vi "ziExample-CNT.vi"() -> ()   [LabVIEW 2009]
doc: "Control a Zurich instrument device via the LabOne Labview API. \nRequirements: Zurich Instruments MFLI, HF2 or UHFLI \nThe example streams the counter data of a trigger input.\n\n© Zurich Instruments AG, www.zhinst.com"
uses:
  <instrlib>/Zurich Instruments LabOne/Public/Configure/ziSetValueDoubleArray.vi
  <instrlib>/Zurich Instruments LabOne/Public/Utility/ziTicksToS_vector.vi
  <instrlib>/Zurich Instruments LabOne/Public/Data/ziGetEventCntSample.vi
  <instrlib>/Zurich Instruments LabOne/Zurich Instruments LabOne.lvlib
panel:
  out "data":cluster{"Timestamp(s)":dbl[], u32[]}
  out "All Values (V)":cluster{"Timestamp(s)":dbl[], i32[]}(graph)
  out "Error Out":errorcluster
  in  "Address":string="DEV"
  out "Selected Device":string
  out "Unexpected Node":string[](array[string])
  in  "stop":bool=TRUE
  # "ziExample-CNT.vi\nRequirements:  UHFLI + CNT Option\nsee block diagram for VI description"
  # "Tested Instruments:\n- UHF"
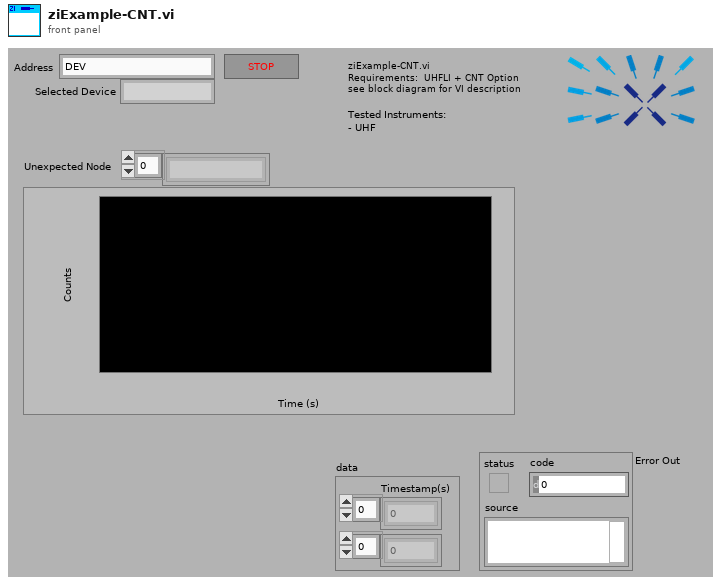
[diagram p1: front panel]
types:
  T1 = typedef "Zurich Instruments LabOne.lvlib/ziTypeHandle.ctl" = cluster{"handleValid":bool, "Conn":u64, "Path Prefix":string, "Handle":u64, "Connected":bool, "Clockbase(s)":dbl}
  T2 = typedef "Zurich Instruments LabOne.lvlib/ziTypeCounterSample.ctl" = cluster{"Timestamps (ticks)":u64[], "Counter":i32[], "Trigger":u32[]}
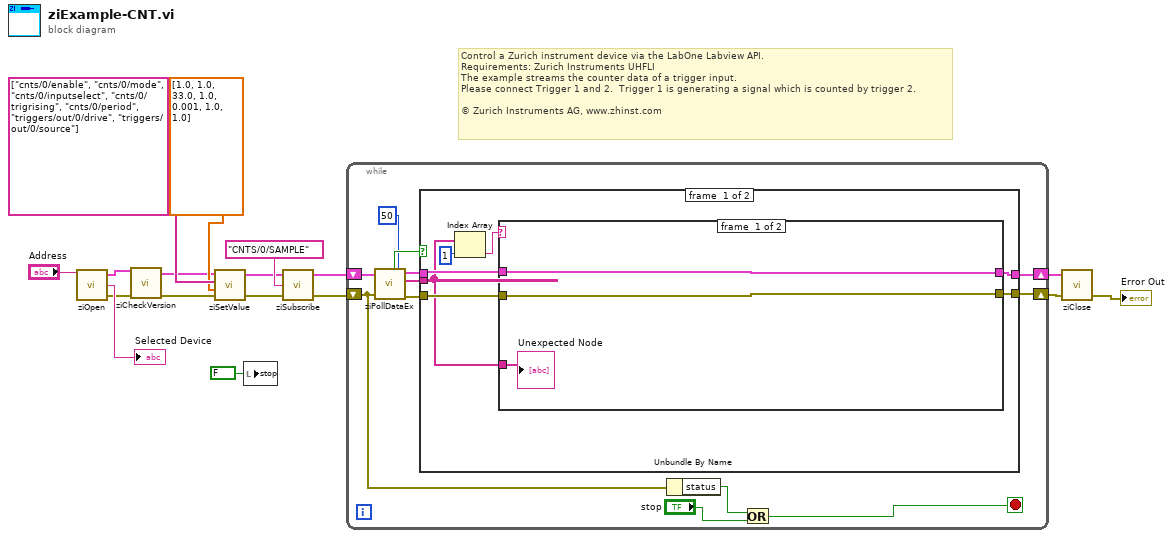
[diagram p0: block diagram]
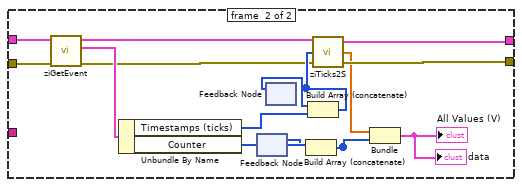
[diagram p2: hidden frame]
diagram:
  # "Control a Zurich instrument device via the LabOne Labview API. \nRequirements: Zurich Instruments UHFLI  \nThe example streams the counter data of a trigger input.\nPlease connect Trigger 1 and 2.  Trigger 1 is generating a signal which is counted by trigger 2.\n\n© Zurich Instruments AG, www.zhinst.com"
  n1 = call <instrlib>:"ziOpen.vi"("Address"="Address") -> ("Error Out"=w3:errorcluster, "Selected Device"=→"Selected Device":string, "HandleOut"=w4:T1)  [unwired: 3 in]
  n2 = call <instrlib>:"ziCheckVersion.vi"("Handle In"=w4, "Error In"=w3) -> ("Handle Out"=w1:T1, "Error Out"=w2:errorcluster)  [unwired: 11 in, 1 out]
  n3 = call-poly <instrlib>:"ziSetValue.vi"("Error In"=w2, "Values"=dbl[] [1.0, 1.0, 33.0, 1.0, 0.001, 1.0, 1.0], "Paths"=string[] ["cnts/0/enable", "cnts/0/mode", "cnts/0/inputselect", "cnts/0/trigrising", "cnts/0/period", "triggers/out/0/drive", "triggers/out/0/source"], "Handle In"=w1) -> ("Error Out"=w6:errorcluster, "Handle Out"=w5:T1)  [unwired: 1 in]
  n4 = local write "stop"(FALSE ("stop")) -> ()
  n5 = call <instrlib>:"ziSubscribe.vi"("error in"=w6, "Path ()"="CNTS/0/SAMPLE", "Handle In"=w5) -> ("error out"=w9:errorcluster, "Handle Out"=w15:T1)  [unwired: 1 in]
  n6 = while {
    shift-right: [w23] -> w16
    shift-left: w15 -> [w29]
    shift-right: [w22] -> w17
    shift-left: w9 -> [w19]
    stop <- w18 stop-if-true
    n7 = call <instrlib>:"ziPollDataEx.vi"("error in"=w19, "Timeout ms (50)"=50 ("TimeOut ms (50)"), "Handle In"=w29) -> ("error out"=w24:errorcluster, "PathArray"=w27:string[], "Handle Out"=w25:T1, "Timed Out"=w28:bool)  [unwired: 1 in, 4 out]
    n8 = case shown="False" w28 {
      tunnel: w27 -> [w30 _]
      tunnel: w25 -> [w36 w56]
      tunnel: w24 -> [w35 w55]
      tunnel: [w34 w56] -> w23
      tunnel: [w33 w55] -> w22
      frame #0 {
        n9 = Index Array(array=w30, index=1) -> (element=w31:string)
        n10 = case shown="\"CNTS\"" w31 {
          tunnel: w36 -> [w39 w54]
          tunnel: w35 -> [w38 w53]
          tunnel: [w39 w45] -> w34
          tunnel: [w38 w43] -> w33
          tunnel: w30 -> [w37 _]
          frame #0 {
            "Unexpected Node" <- w37
          }
          frame #1 {
            n11 = call-poly <instrlib>:"ziGetEvent.vi"("Error In"=w53, "Handle In"=w54) -> ("Error Out"=w44:errorcluster, "Cnt Sample Out"=w52:T2, "Handle Out"=w46:T1)  [unwired: 7 in]
            n12 = Unbundle By Name(w52) -> ("Timestamps (ticks)"=w51:u64[], "Counter"=w49:i32[])
            n13 = feedback #1() -> (w48:i32[])  [unwired: 1 in]
            n14 = feedback #2() -> (w50:u64[])  [unwired: 1 in]
            n15 = Build Array (concatenate)(w48, w49) -> (w42:i32[])
            n16 = Build Array (concatenate)(w50, w51) -> (w47:u64[])
            n17 = call-poly <instrlib>:"ziTicks2S.vi"("Error In"=w44, "Timestamp (ticks)"=w47, "Handle In"=w46) -> ("Error Out"=w43:errorcluster, "Timestamp(s)"=w41:dbl[], "Handle Out"=w45:T1)
            n18 = Bundle("Timestamp(s)"=w41, w42) -> (→"All Values (V)" →"data":cluster{"Timestamp(s)":dbl[], i32[]})  [unwired: 1 in]
          }
        }
      }
      frame #1 {
      }
    }
    n19 = Unbundle By Name(w19) -> ("status"=w21:bool)
    n20 = Or(x=w21, y="stop") -> (x .or. y?=w18:bool)
  }
  n21 = call <instrlib>:"ziClose.vi"("Error In"=w17, "Handle In"=w16) -> ("Error Out"=→"Error Out":errorcluster)  [unwired: 2 in, 1 out]
